vi "Process UDP Input.vi"(8 "error in (no error)":errorcluster, 11 "UDP Network Connection in":refnum<k16>) -> (0 "error out":errorcluster, 2 "Data From XPlane":sgl[](array[numeric]), 3 "UDP Network Connection out":refnum<k16>)   [LabVIEW 2014]
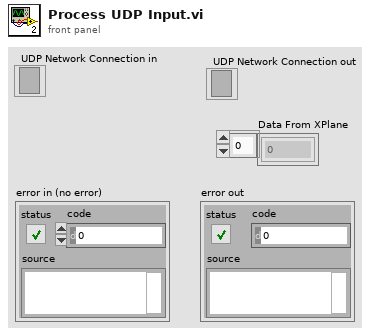
[diagram p1: front panel]
types:
  T1 = cluster{sgl, sgl, sgl, sgl, sgl, sgl, sgl, sgl, sgl, sgl, sgl, sgl, sgl, sgl, sgl, sgl, sgl, sgl, sgl, sgl, sgl, sgl, sgl, sgl, sgl, sgl, sgl, sgl, sgl, sgl, sgl, sgl, sgl, sgl, sgl, sgl}
  T2 = enum16{"big-endian, network order", "native, host order", "little-endian"}
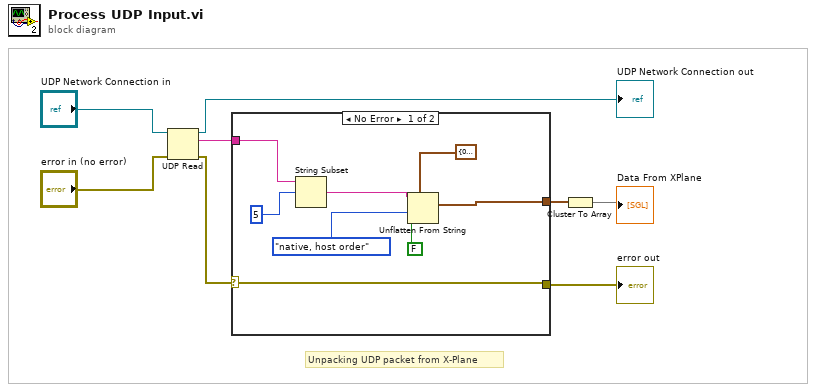
[diagram p0: block diagram]
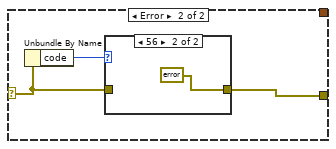
[diagram p2: hidden frame]
diagram:
  # "Unpacking UDP packet from X-Plane"
  n1 = UDP Read(connection ID="UDP Network Connection in", 8:"error in (no error)") -> (data out=w6:string, error out=w7:errorcluster, 3:→"UDP Network Connection out":refnum<k16>)  [unwired: 2 in, 2 out]
  n2 = case shown="No Error" w7 {
    selector: w7 -> [w9 w18]
    tunnel: w6 -> [w16 _]
    tunnel: [w10 _] -> w2
    tunnel: [w9 w17] -> w8
    frame No Error {
      n3 = String Subset(string=w16, offset (0)=5) -> (substring=w12:string)  [unwired: 1 in]
      n4 = Unflatten From String(type=T1 {0.0, 0.0, 0.0, 0.0, 0.0, 0.0, 0.0, 0.0, 0.0, 0.0, 0.0, 0.0, 0.0, 0.0, 0.0, 0.0, 0.0, 0.0, 0.0, 0.0, 0.0, 0.0, 0.0, 0.0, 0.0, 0.0, 0.0, 0.0, 0.0, 0.0, 0.0, 0.0, 0.0, 0.0, 0.0, 0.0}, binary string=w12, data includes array or string size? (T)=FALSE, byte order (0:big-endian, network order)=T2."native, host order") -> (value=w10:T1)  [unwired: 1 in, 2 out]
    }
    frame Error {
      n5 = Unbundle By Name(w18) -> ("code"=w19:i32)
      n6 = case shown="56" w19 {
        tunnel: w18 -> [w20 _]
        tunnel: [w20 errorcluster {"status"=FALSE, "code"=0, "source"=""} ("error IO")] -> w17
        frame 0, Default {
        }
        frame 56 {
        }
      }
    }
  }
  "error out" <- w8
  n7 = Cluster To Array(cluster=w2) -> (array=→"Data From XPlane":sgl[])
